vi "Event Read Symbol.vi"() -> ()   [LabVIEW 2018]
uses:
  TwinCAT ADS Class/Controls/Symbol Information.ctl
  TwinCAT ADS Class/TwinCAT ADS.lvclass/TwinCAT ADS.ctl
  TwinCAT ADS Class/VIs/Delete Notification From Map.vi
  TwinCAT ADS Class/VIs/Get Notification Map.vi
  TwinCAT ADS Class/VIs/To Notification Key.vi
  <vilib>/Utility/error.llb/Trim Whitespace.vi
  TwinCAT ADS Class/VIs/Extensions/Delete Notification By Handle.vi
  TwinCAT ADS Class/TwinCAT ADS.lvclass
panel:
  out "Alias":string
  in  "Cycle Time (ms)":i32=60
  in  "Alias":string
  in  "Symbol Name":string="MAIN.arstCat"
  in  "Remove Symbol":bool
  in  "Add Symbol":bool
  in  "Stop":bool
  out "Value":variant=variant(cluster{bool, bool, sgl}[] [{FALSE, FALSE, 0.0}, {FALSE, FALSE, 0.0}, {FALSE, FALSE, 0.0}, {FALSE, FALSE, 0.0}, {FALSE, FALSE, 0.0}, {FALSE, FALSE, 0.0}, {TRUE, FALSE, 0.0}, {FALSE, FALSE, 0.0}, {FALSE, FALSE, 0.0}, {FALSE, FALSE, 0.0}, {FALSE, FALSE, 0.0}, {FALSE, FALSE, 0.0}, {FALSE, FALSE, 0.0}, {FALSE, FALSE, 0.0}, {FALSE, FALSE, 0.0}, {FALSE, FALSE, 0.0}, {FALSE, FALSE, 0.0}, {FALSE, FALSE, 0.0}, {FALSE, FALSE, 0.0}, {FALSE, FALSE, 0.0}, {FALSE, FALSE, 0.0}, {FALSE, FALSE, 0.0}, {FALSE, FALSE, 0.0}, {FALSE, FALSE, 0.0}, {FALSE, FALSE, 0.0}, {FALSE, FALSE, 0.0}, {FALSE, FALSE, 0.0}, {FALSE, FALSE, 0.0}, {FALSE, FALSE, 0.0}, {FALSE, FALSE, 0.0}, {FALSE, FALSE, 0.0}, {FALSE, FALSE, 0.0}, {FALSE, FALSE, 0.0}, {FALSE, FALSE, 0.0}, {FALSE, FALSE, 0.0}, {FALSE, FALSE, 0.0}, {FALSE, FALSE, 0.0}, {FALSE, FALSE, 0.0}, {FALSE, FALSE, 0.0}, {FALSE, FALSE, 0.0}, {FALSE, FALSE, 0.0}, {FALSE, FALSE, 0.0}, {FALSE, FALSE, 0.0}, {FALSE, FALSE, 0.0}, {FALSE, FALSE, 0.0}, {FALSE, FALSE, 0.0}, {FALSE, FALSE, 0.0}, {FALSE, FALSE, 0.0}, {FALSE, FALSE, 0.0}, {FALSE, FALSE, 0.0}, {FALSE, FALSE, 0.0}, {FALSE, FALSE, 0.0}, {FALSE, FALSE, 0.0}, {FALSE, FALSE, 0.0}, {FALSE, FALSE, 0.0}, {FALSE, FALSE, 0.0}, {FALSE, FALSE, 0.0}, {FALSE, FALSE, 0.0}, {FALSE, FALSE, 0.0}, {FALSE, FALSE, 0.0}, {FALSE, FALSE, 0.0}, {FALSE, FALSE, 0.0}, {FALSE, FALSE, 0.0}, {FALSE, FALSE, 0.0}, {FALSE, FALSE, 0.0}, {FALSE, FALSE, 0.0}, {FALSE, FALSE, 0.0}, {FALSE, FALSE, 0.0}, {FALSE, FALSE, 0.0}, {FALSE, FALSE, 0.0}, {FALSE, FALSE, 0.0}, {FALSE, FALSE, 0.0}, {FALSE, FALSE, 0.0}, {FALSE, FALSE, 0.0}, {FALSE, FALSE, 0.0}, {FALSE, FALSE, 0.0}, {FALSE, FALSE, 0.0}, {FALSE, FALSE, 0.0}, {FALSE, FALSE, 0.0}, {FALSE, FALSE, 0.0}, {FALSE, FALSE, 0.0}, {FALSE, FALSE, 0.0}, {FALSE, FALSE, 0.0}, {FALSE, FALSE, 0.0}, {FALSE, FALSE, 0.0}, {FALSE, FALSE, 0.0}, {FALSE, FALSE, 0.0}, {FALSE, FALSE, 0.0}, {FALSE, FALSE, 0.0}, {FALSE, FALSE, 0.0}, {FALSE, FALSE, 0.0}, {FALSE, FALSE, 0.0}, {FALSE, FALSE, 0.0}, {FALSE, FALSE, 0.0}, {FALSE, FALSE, 0.0}, {FALSE, FALSE, 0.0}, {FALSE, FALSE, 0.0}, {FALSE, FALSE, 0.0}, {FALSE, FALSE, 0.0}, {FALSE, FALSE, 0.0}])
  out "Symbol Info":T1={"Name"="MAIN.arstCat", "Short Name"="MAIN.arstCat", "Size"=800, "Type Category"=4, "Type Name"="ARRAY [0..99] OF ST_CAT", "Type ID"=65, "Index Group"=16448, "Index Offset"=396892, "Child Count"=100, "Has Rpc Methods?"=FALSE, "Comment"=""} {"Type ID" items=["ADST_VOID"=0, "ADST_INT16"=2, "ADST_INT32"=3, "ADST_REAL32"=4, "ADST_REAL64"=5, "ADST_INT8"=16, "ADST_UINT8"=17, "ADST_UINT16"=18, "ADST_UINT32"=19, "ADST_INT64"=20, "ADST_UINT64"=21, "ADST_STRING"=30, "ADST_WSTRING"=31, "ADST_REAL80"=32, "ADST_BIT"=33, "ADST_MAXTYPES"=34, "ADST_BIGTYPE"=65]; "Type Category" items=["Unknown, None"=0, "Primitive"=1, "Alias"=2, "Enum"=3, "Array"=4, "Struct"=5, "FunctionBlock"=6, "Program"=7, "Function"=8, "SubRange"=9, "String"=10, "Bitset"=12, "Pointer"=13, "Union"=14, "Reference"=15, "Interface"=16]}
  # "Example PLC Source Code is available at:\nhttps://github.com/fisothemes/LabVIEW-TwinCAT-ADS/tree/master/src/PLC"
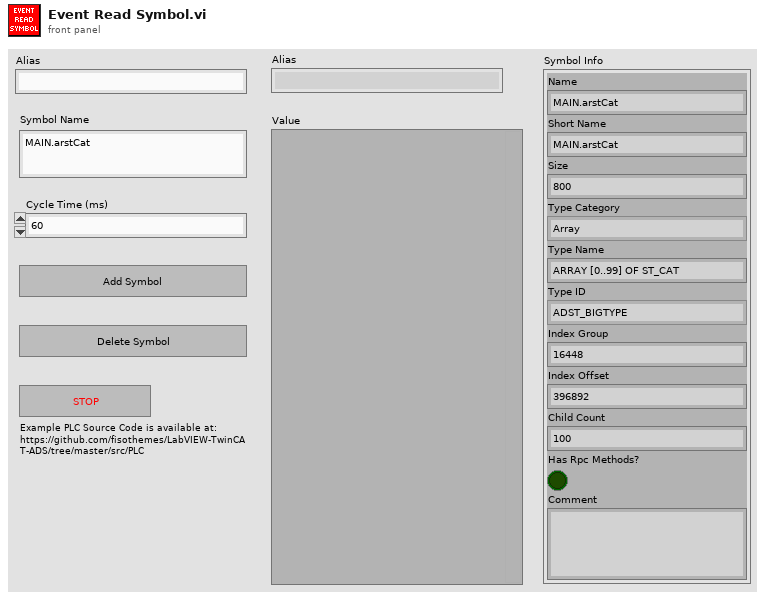
[diagram p1: front panel]
types:
  T1 = typedef "TwinCAT ADS.lvclass/Symbol Information.ctl" = cluster{"Name":string, "Short Name":string, "Size":i32, "Type Category":i32, "Type Name":string, "Type ID":i32, "Index Group":i64, "Index Offset":i64, "Child Count":i32, "Has Rpc Methods?":bool, "Comment":string}
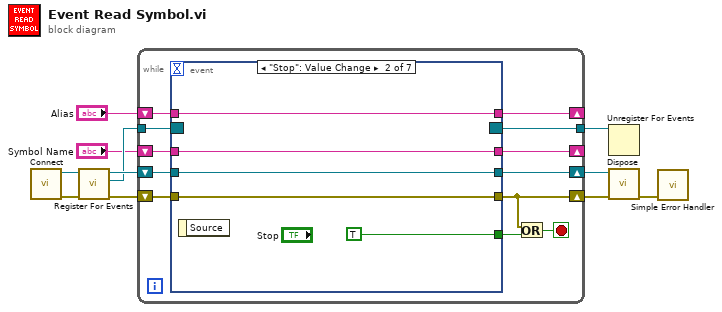
[diagram p0: block diagram]
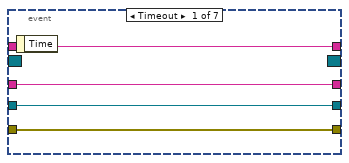
[diagram p2: hidden frame]
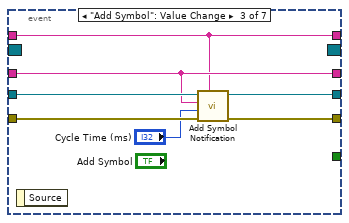
[diagram p3: hidden frame]
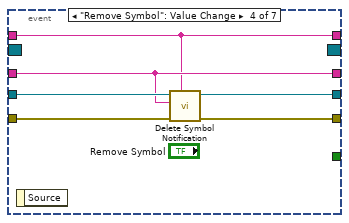
[diagram p4: hidden frame]
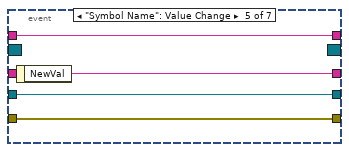
[diagram p5: hidden frame]
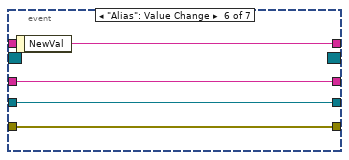
[diagram p6: hidden frame]
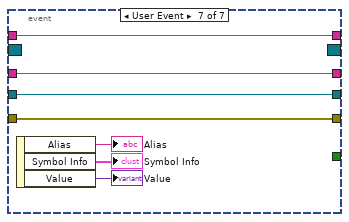
[diagram p7: hidden frame]
diagram:
  n1 = call "Connect.vi"() -> ("error out"=w10:errorcluster, "TwinCAT ADS out"=w11:refnum<class "TwinCAT ADS.lvclass">)  [unwired: 10 in]
  n2 = call "Register For Events.vi"("error in (no error)"=w10, "TwinCAT ADS in"=w11) -> ("error out"=w8:errorcluster, "Event Registration Refnum"=w3:refnum<event-registration>, "TwinCAT ADS out"=w9:refnum<class "TwinCAT ADS.lvclass">)  [unwired: 7 in]
  n3 = while {
    shift-right: [w21] -> w7
    shift-left: w9 -> [w23]
    shift-right: [w20] -> w6
    shift-left: w8 -> [w22]
    tunnel: w3 -> [w17]
    tunnel: [w16] -> w4
    shift-right: [w15] -> _
    shift-left: "Symbol Name" -> [w14]
    shift-right: [w12] -> _
    shift-left: "Alias" -> [w13]
    stop <- w18 stop-if-true
    n4 = event shown="[1] \"Stop\": Value Change" {
      selector: w17 -> [_ _ _ _ _ _ _]
      dyn-events: [_ _ _ _ _ _ _] -> w16
      timeout: _ -> [_ _ _ _ _ _ _]
      tunnel: w23 -> [w27 w32 w39 w45 w49 w53 w60]
      tunnel: w22 -> [w26 w31 w38 w44 w48 w52 w59]
      tunnel: [w27 w32 w36 w42 w49 w53 w60] -> w21
      tunnel: [w26 w31 w35 w43 w48 w52 w59] -> w20
      tunnel: [_ TRUE _ _ _ _ _] -> w19
      tunnel: [w25 w29 w37 w41 w47 w51 w58] -> w15
      tunnel: w14 -> [w25 w29 w37 w41 _ w51 w58]
      tunnel: w13 -> [w24 w28 w33 w40 w46 _ w55]
      tunnel: [w24 w28 w33 w40 w46 w50 w55] -> w12
      event Timeout {
        n5 = event-data() -> ()  [unwired: 1 in, 1 out]
      }
      event "Stop": Value Change {
        n6 = event-data() -> ()  [unwired: 1 in, 1 out]
      }
      event "Add Symbol": Value Change {
        n7 = event-data() -> ()  [unwired: 1 in, 1 out]
        n8 = call "Add Symbol Notification.vi"("Alias"=w33, "error in (no error)"=w38, "Cycle Time (ms)"="Cycle Time (ms)", "Symbol Name"=w37, "TwinCAT ADS in"=w39) -> ("error out"=w35:errorcluster, "TwinCAT ADS out"=w36:refnum<class "TwinCAT ADS.lvclass">)  [unwired: 5 in]
      }
      event "Remove Symbol": Value Change {
        n9 = event-data() -> ()  [unwired: 1 in, 1 out]
        n10 = call "Delete Symbol Notification.vi"("Alias"=w40, "error in (no error)"=w44, "Symbol Name"=w41, "TwinCAT ADS in"=w45) -> ("error out"=w43:errorcluster, "TwinCAT ADS out"=w42:refnum<class "TwinCAT ADS.lvclass">)  [unwired: 6 in]
      }
      event "Symbol Name": Value Change {
        n11 = event-data() -> ("NewVal"=w47:string)  [unwired: 1 in]
      }
      event "Alias": Value Change {
        n12 = event-data() -> ("NewVal"=w50:string)  [unwired: 1 in]
      }
      event User Event {
        n13 = event-data() -> ("Alias"=→"Alias":string, "Symbol Info"=→"Symbol Info":T1, "Value"=→"Value":variant)  [unwired: 1 in]
      }
    }
    n14 = Or(x=w20, y=w19) -> (x .or. y?=w18:bool)
  }
  n15 = Unregister For Events(event registration refnum=w4) -> ()  [unwired: 1 in, 1 out]
  n16 = call "Dispose.vi"("error in (no error)"=w6, "TwinCAT ADS in"=w7) -> ("error out"=w5:errorcluster)  [unwired: 9 in]
  n17 = call <vilib>:"Simple Error Handler.vi"("error in (no error)"=w5) -> ()  [unwired: 4 in, 5 out]
